vi "Joystick - Close All.vi"() -> ()   [LabVIEW 2015]
uses:
  <vilib>/Rock Robotics/WPI/Utilities/WPI_GetSetVariantRefNum.vi
panel:
  out "error out":errorcluster
  in  "error in (no error)":errorcluster
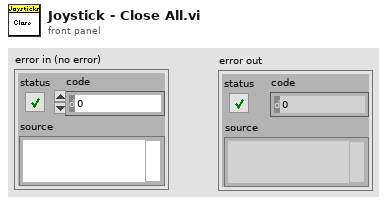
[diagram p1: front panel]
types:
  T1 = typedef "WPI_JoystickDevRef.ctl" = cluster{"Device":T2}
  T2 = typedef "WPI_JoystickDeviceEnum.ctl" = enum16{"USB 0", "USB 1", "USB 2", "USB 3", "USB 4", "USB 5"}
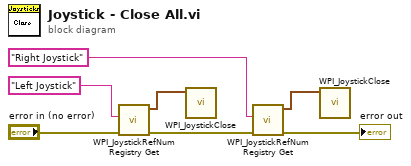
[diagram p0: block diagram]
diagram:
  n1 = call <vilib>:"WPI_JoystickRefNum Registry Get.vi"("error in (no error)"="error in (no error)", "refnum name"="Left Joystick") -> ("error out"=w3:errorcluster, "JoystickDevRef"=w4:T1)  [unwired: 8 in]
  n2 = call <vilib>:"WPI_JoystickClose.vi"("JoystickDevRef"=w4) -> ()  [unwired: 11 in]
  n3 = call <vilib>:"WPI_JoystickRefNum Registry Get.vi"("error in (no error)"=w3, "refnum name"="Right Joystick") -> ("error out"=→"error out":errorcluster, "JoystickDevRef"=w5:T1)  [unwired: 8 in]
  n4 = call <vilib>:"WPI_JoystickClose.vi"("JoystickDevRef"=w5) -> ()  [unwired: 11 in]
